vi "scrollbar_index-point.vi"(8 "error in (no error)":errorcluster, 9 "seek":i32, 10 "data_display":i32, 11 "data_available":i32) -> (0 "error out":errorcluster, 2 "length":i32=-1, 3 "index":i32=-1)   [LabVIEW 2015, in "lv-graph.lvlib"]
doc: "This VI will relegate scrollbar values with the data available and what's visible on the graph."
uses:
  lv-graph.lvlib
panel:
  in  "use_multiplier":bool
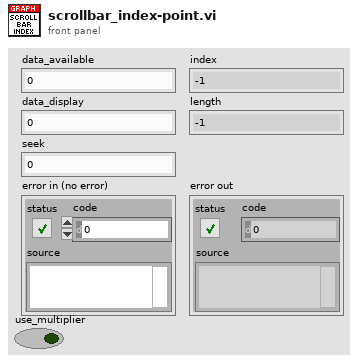
[diagram p1: front panel]
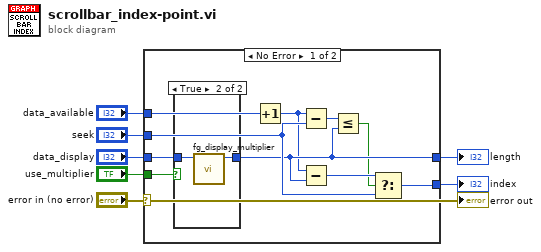
[diagram p0: block diagram]
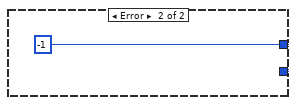
[diagram p3: hidden frame]
diagram:
  n1 = case shown="No Error" "error in (no error)" {
    tunnel: "seek" -> [w17 _]
    tunnel: "data_display" -> [w16 _]
    tunnel: [w15 w21] -> w5
    tunnel: [w14 w21] -> w4
    tunnel: "data_available" -> [w13 _]
    tunnel: "use_multiplier" -> [w8 _]
    frame No Error {
      n2 = case shown="True" w8 {
        tunnel: w16 -> [w18 w19]
        tunnel: [w18 w20] -> w14
        frame False {
        }
        frame True {
          n3 = call "fg_display_multiplier.vi"("n_data in"=w19) -> ("n_data out"=w20:i32)  [unwired: 9 in, 1 out]
        }
      }
      n4 = Increment(x=w13) -> (x+1=w12:i32)
      n5 = Subtract(x=w12, y=w17) -> (x-y=w11:i32)
      n6 = Subtract(x=w12, y=w14) -> (x-y=w10:i32)
      n7 = Less Or Equal?(x=w11, y=w14) -> (x <= y?=w9:bool)
      n8 = Select(t=w10, s=w9, f=w17) -> (s? t:f=w15:i32)
    }
    frame Error {
      w21 = -1 ("Seek")
    }
  }
  "index" <- w5
  "length" <- w4
  "error out" <- "error in (no error)"
